vi "Setup Statically-Linked subWorkers.vi"(8 "error in":errorcluster, 11 "ChartView in":refnum<class "ChartView.lvclass">) -> (0 "error out":errorcluster, 3 "ChartView out":refnum<class "ChartView.lvclass">)   [LabVIEW 2020, in "ChartView.lvclass"]
doc: "This VI performs a setup of all the statically-linked subWorkers that belong to the Worker that owns this VI. This VI must be called <b>before</b> any statically-linked subWorkers are called."
uses:
  ChartView.lvclass
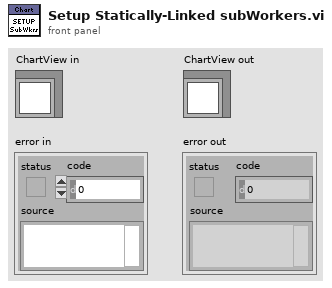
[diagram p1: front panel]
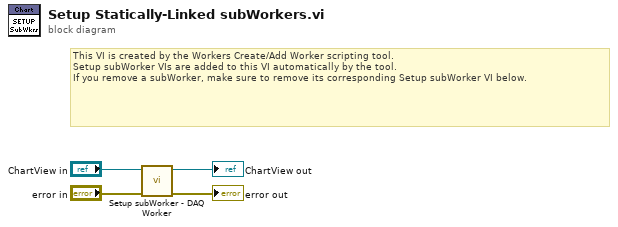
[diagram p0: block diagram]
diagram:
  # "This VI is created by the Workers Create/Add Worker scripting tool.\nSetup subWorker VIs are added to this VI automatically by the tool.\nIf you remove a subWorker, make sure to remove its corresponding Setup subWorker VI below."
  n1 = call "Setup subWorker - DAQ Worker.vi"("error in"="error in", "ChartView in"="ChartView in") -> ("error out"=→"error out":errorcluster, "ChartView out"=→"ChartView out":refnum<class "ChartView.lvclass">)  [unwired: 8 in]
